vi "Set Point.vi"(8 "error in (no error)":errorcluster, 10 "Set point":dbl, 11 "LakeShore T Controller Driver in":refnum<class "LakeShore T Controller Driver.lvclass">) -> (0 "error out":errorcluster, 3 "LakeShore T Controller Driver out":refnum<class "LakeShore T Controller Driver.lvclass">)   [LabVIEW 2016, in "LakeShore T Controller Driver.lvclass"]
uses:
  LakeShore T Controller Driver.lvclass
  C:/github/NHMFL_Core/Libraries/Instruments/VISA Instrument/VISA Instrument.lvclass
  VISA Instrument/VISA Instrument.lvclass/VISA Instrument.ctl
  VISA Instrument/Read VISA resource.vi
  VISA Instrument/Write VISA resource.vi
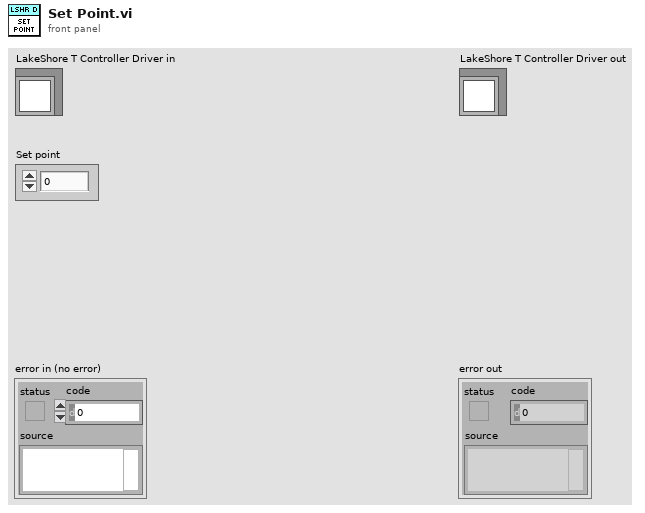
[diagram p1: front panel]
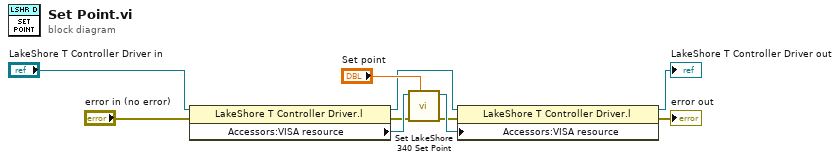
[diagram p0: block diagram]
diagram:
  n1 = property class="LakeShore T Controller Driver.l"(reference="LakeShore T Controller Driver in", error in="error in (no error)") -> (reference out=w1:refnum<class "LakeShore T Controller Driver.lvclass">, error out=w2:errorcluster, "Accessors:VISA resource"=w9:refnum<visa-resource-name>)
  n2 = call "Set LakeShore 340 Set Point.vi"("Set point"="Set point", "error in (no error)"=w2, "VISA Resource Name"=w9) -> ("error out"=w5:errorcluster, "VISA Resource Name Out"=w6:refnum<visa-resource-name>)  [unwired: 7 in]
  n3 = property class="LakeShore T Controller Driver.l"(reference=w1, error in=w5, "Accessors:VISA resource"=w6) -> (reference out=→"LakeShore T Controller Driver out":refnum<class "LakeShore T Controller Driver.lvclass">, error out=→"error out":errorcluster)
